vi "closeFile.vi"(8 "error in (no error)":errorcluster, 11 "Handler.File in":refnum<class "Handler.File.lvclass">) -> (0 "error out":errorcluster, 3 "Handler.File out":refnum<class "Handler.File.lvclass">)   [LabVIEW 2017, in "Error Log.lvlib" / "Handler.File.lvclass"]
uses:
  Handler.File.lvclass
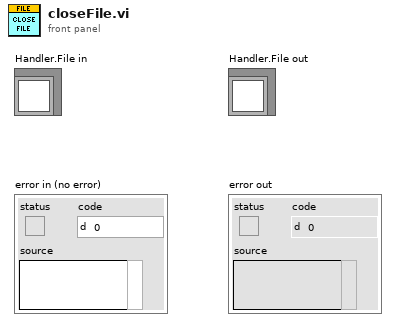
[diagram p1: front panel]
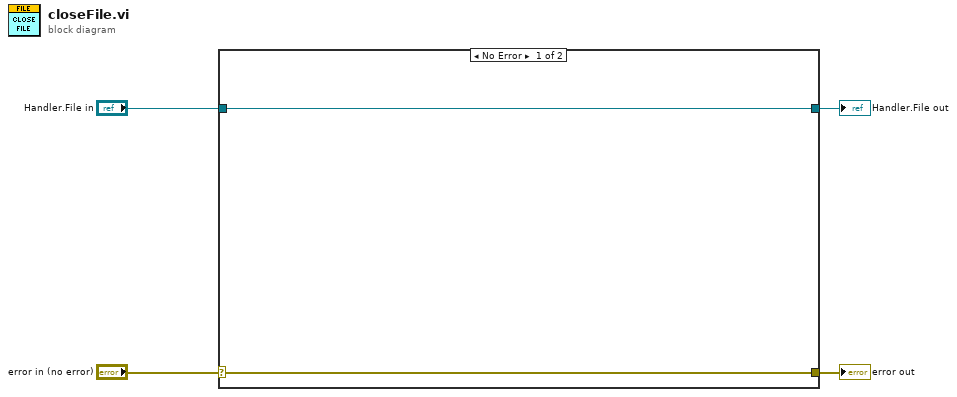
[diagram p0: block diagram]
diagram:
  n1 = case shown="No Error" "error in (no error)" {
    selector: "error in (no error)" -> [w5 w8]
    tunnel: [w5 w8] -> w3
    tunnel: [w6 w7] -> w1
    tunnel: "Handler.File in" -> [w6 w7]
    frame No Error {
    }
    frame Error {
    }
  }
  "error out" <- w3
  "Handler.File out" <- w1
